vi "host_form_list.vi"() -> (2 "paths":path[](array[path]), 3 "names":string[](array[string]))   [LabVIEW 2021]
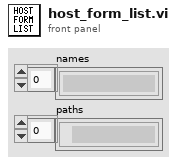
[diagram p1: front panel]
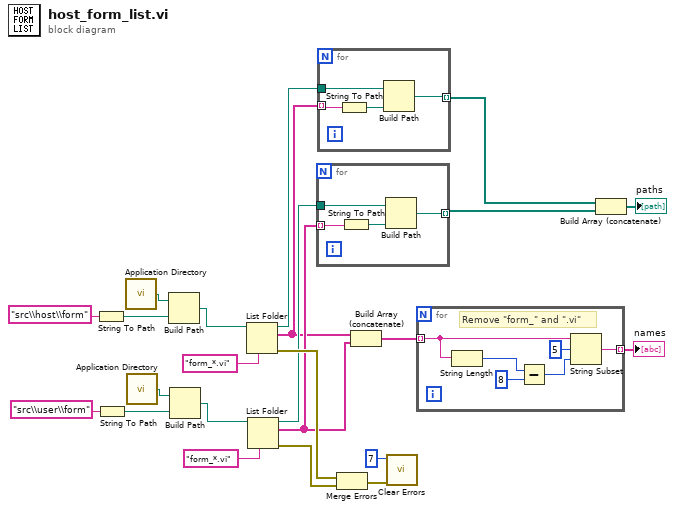
[diagram p0: block diagram]
diagram:
  n1 = String To Path(string="src\\host\\form") -> (path=w21:path)
  n2 = String To Path(string="src\\user\\form") -> (path=w16:path)
  n3 = call <vilib>:"Application Directory.vi"() -> ("Application Directory"=w23:path)
  n4 = call <vilib>:"Application Directory.vi"() -> ("Application Directory"=w14:path)
  n5 = Build Path(base path=w23, name or relative path=w21) -> (appended path=w20:path)
  n6 = Build Path(base path=w14, name or relative path=w16) -> (appended path=w17:path)
  n7 = List Folder(path=w20, pattern="form_*.vi") -> (path out=w7:path, filenames=w4:string[], error out=w10:errorcluster)  [unwired: 2 in, 1 out]
  n8 = List Folder(path=w17, pattern="form_*.vi") -> (path out=w6:path, filenames=w5:string[], error out=w9:errorcluster)  [unwired: 2 in, 1 out]
  n9 = for {
    tunnel: w6 -> [w25]
    tunnel: w5 -> [w26] mode=indexing
    tunnel: [w24] -> w2 mode=indexing
    n10 = String To Path(string=w26) -> (path=w27:path)
    n11 = Build Path(base path=w25, name or relative path=w27) -> (appended path=w24:path)
  }
  n12 = for {
    tunnel: w7 -> [w29]
    tunnel: w4 -> [w31] mode=indexing
    tunnel: [w28] -> w3 mode=indexing
    n13 = String To Path(string=w31) -> (path=w30:path)
    n14 = Build Path(base path=w29, name or relative path=w30) -> (appended path=w28:path)
  }
  n15 = Merge Errors(w10, w9) -> (w11:errorcluster)
  n16 = Build Array (concatenate)(w4, w5) -> (w13:string[])
  n17 = call <vilib>:"Clear Errors.vi"("error in (no error)"=w11, "specific error code to clear (0: all)"=7) -> ()  [unwired: 4 in, 2 out]
  n18 = for {
    tunnel: w13 -> [w33] mode=indexing
    tunnel: [w32] -> w12 mode=indexing
    # "Remove \"form_\" and \".vi\""
    n19 = String Length(string=w33) -> (length=w35:i32)
    n20 = Subtract(x=w35, y=8) -> (x-y=w36:i32)
    n21 = String Subset(string=w33, offset (0)=5, length (rest)=w36) -> (substring=w32:string)
  }
  "names" <- w12
  n22 = Build Array (concatenate)(w3, w2) -> (→"paths":path[])
